vi "fgv_reg_test-specs.vi"(7 "cmd":T2, 11 "고장진단 기준 값":T1 {"출력단 특성전류 Irms[mA]  Min" format="%#.2f"; "출력단 특성 전류 Irms[mA]  Max" format="%#.2f"; "출력단 단선 Irms[mA](이하)" format="%#.2f"; "제어단 특성 전류 Irms[mA] Min" format="%#.2f"; "제어단 특성 전류 Irms[mA] Max" format="%#.2f"; "제어단 단선 Irms[mA](이하)" format="%#.2f"}) -> (3 "고장진단 기준 값 2":T1 {"출력단 특성전류 Irms[mA]  Min" format="%#.2f"; "출력단 특성 전류 Irms[mA]  Max" format="%#.2f"; "출력단 단선 Irms[mA](이하)" format="%#.2f"; "제어단 특성 전류 Irms[mA] Min" format="%#.2f"; "제어단 특성 전류 Irms[mA] Max" format="%#.2f"; "제어단 단선 Irms[mA](이하)" format="%#.2f"})   [LabVIEW 2019]
uses:
  _ctrl/rw.ctl
  Breakdown-Spec.ctl
panel:
  # "제어단"
  # "출력단"
  # "온도기준"
  # "제어단"
  # "출력단"
  # "온도기준"
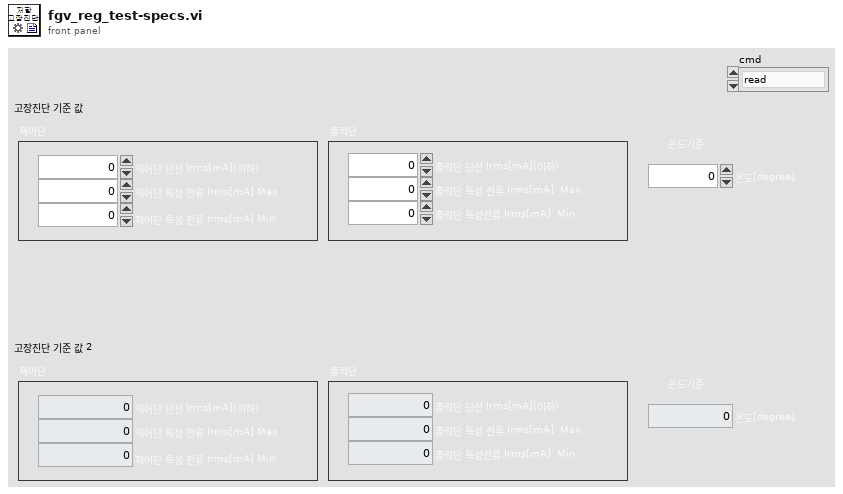
[diagram p1: front panel]
types:
  T1 = typedef "Breakdown-Spec.ctl" = cluster{"제어단 단선 Irms[mA](이하)":dbl, "제어단 특성 전류 Irms[mA] Max":dbl, "제어단 특성 전류 Irms[mA] Min":dbl, "출력단 단선 Irms[mA](이하)":dbl, "출력단 특성 전류 Irms[mA]  Max":dbl, "출력단 특성전류 Irms[mA]  Min":dbl, "온도[degree]":dbl}
  T2 = typedef "rw.ctl" = enum16{"read", "write"}
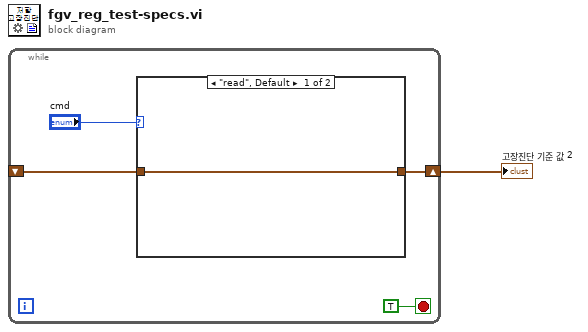
[diagram p0: block diagram]
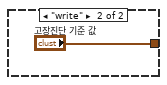
[diagram p2: hidden frame]
diagram:
  n1 = while {
    shift-right: [w3] -> w1
    shift-left: _ -> [w2]
    stop <- TRUE stop-if-true
    n2 = case shown="\"read\", Default" "cmd" {
      tunnel: [w6 "고장진단 기준 값"] -> w3
      tunnel: w2 -> [w6 _]
      frame "read", Default {
      }
      frame "write" {
      }
    }
  }
  "고장진단 기준 값 2" <- w1
